vi "Programmatically Save Control Values 86 Updated 2016 09 for LV12.vi"() -> ()   [LabVIEW 2012]
panel:
  in  "Numeric 2":dbl
  in  "STOP":bool
  in  "String":string="test"
  in  "Boolean 2":bool=TRUE
  in  "Numeric":dbl=35.0
  in  "Boolean":bool=TRUE
  in  "LOAD":bool
  in  "SAVE":bool
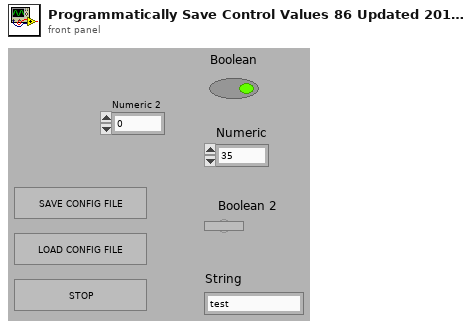
[diagram p1: front panel]
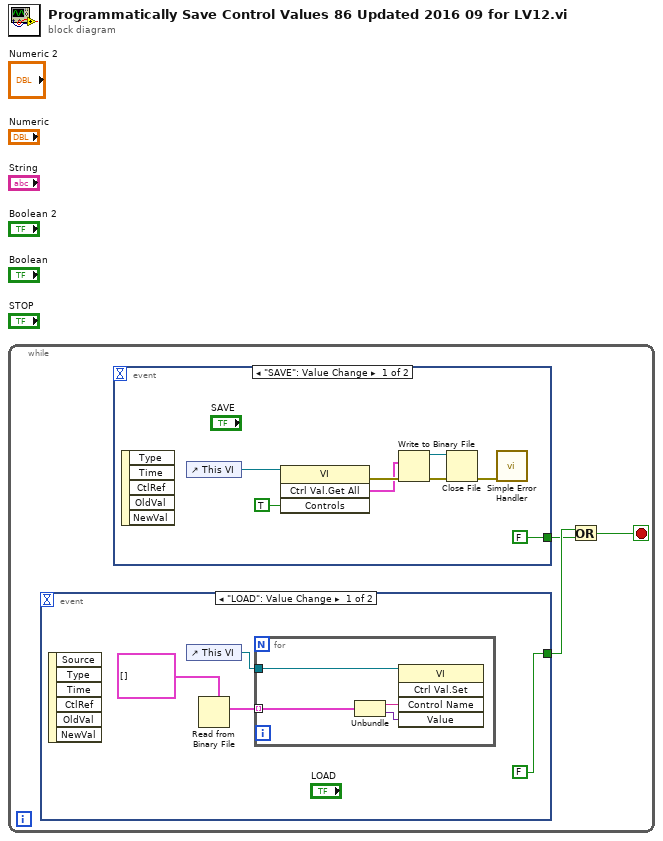
[diagram p0: block diagram]
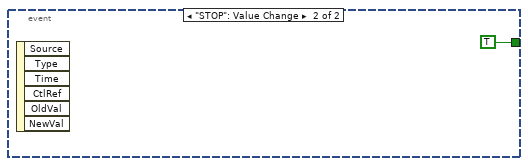
[diagram p2: hidden frame]
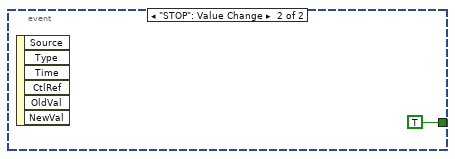
[diagram p3: hidden frame]
diagram:
  n1 = while {
    stop <- w2 stop-if-true
    n2 = event shown="[0] \"LOAD\": Value Change" {
      selector: _ -> [_ _]
      dyn-events: _ -> [_ _]
      timeout: _ -> [_ _]
      tunnel: [FALSE TRUE] -> w3
      event "LOAD": Value Change {
        n3 = event-data() -> ()  [unwired: 7 out]
        n4 = control-ref of="This VI"() -> (w7:refnum<vi>)
        n5 = Read from Binary File(5:cluster{"Name":string, "Variant Data":variant}[] [] ("Control Value:Get All")) -> (2:w4:cluster{"Name":string, "Variant Data":variant}[])  [unwired: 5 in, 3 out]
        n6 = for {
          tunnel: w7 -> [w11]
          tunnel: w4 -> [w10] mode=indexing
          n7 = Unbundle(w10) -> ("Name"=w9:string, "Variant Data"=w8:variant)
          n8 = invoke class="VI" method="Ctrl Val.Set"(reference=w11, "Control Name"=w9, "Value"=w8) -> ()  [unwired: 2 in, 5 out]
        }
      }
      event "STOP": Value Change {
        n9 = event-data() -> ()  [unwired: 7 out]
      }
    }
    n10 = event shown="[0] \"SAVE\": Value Change" {
      selector: _ -> [_ _]
      dyn-events: _ -> [_ _]
      timeout: _ -> [_ _]
      tunnel: [FALSE TRUE] -> w1
      event "SAVE": Value Change {
        n11 = event-data() -> ()  [unwired: 6 out]
        n12 = control-ref of="This VI"() -> (w19:refnum<vi>)
        n13 = invoke class="VI" method="Ctrl Val.Get All"(reference=w19, "Controls"=TRUE) -> (error out=w16:errorcluster, "Get All Control Values Variant"=w15:cluster{"Name":string, "Variant Data":variant}[])  [unwired: 2 in, 2 out]
        n14 = Write to Binary File(data=w15, error in=w16) -> (refnum out=w13:refnum<file>, error out=w14:errorcluster)  [unwired: 4 in, 1 out]
        n15 = Close File(refnum=w13, error in=w14) -> (error out=w18:errorcluster)  [unwired: 1 out]
        n16 = call <vilib>:"Simple Error Handler.vi"("error in (no error)"=w18) -> ()  [unwired: 1 in, 8 out]
      }
      event "STOP": Value Change {
        n17 = event-data() -> ()  [unwired: 7 out]
      }
    }
    n18 = Or(x=w3, y=w1) -> (x .or. y?=w2:bool)
  }
